vi "Track Rotation.vi"(8 "Angle Limiter":enum16{"90", "45", "15", "1"}(ring), 10 "Coord":cluster{dbl, dbl}, 11 "Point in":cluster{"x":dbl, "y":dbl, "th":dbl}) -> (3 "Point out":cluster{"x":dbl, "y":dbl, "th":dbl})   [LabVIEW 2018]
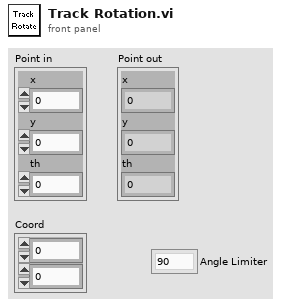
[diagram p1: front panel]
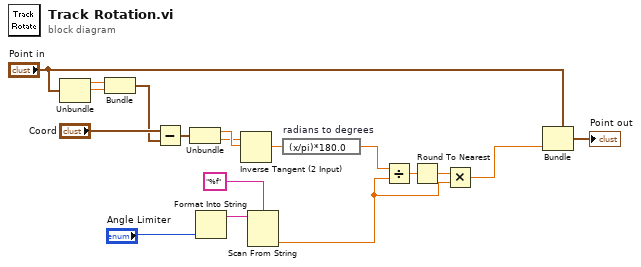
[diagram p0: block diagram]
diagram:
  n1 = Unbundle("Point in") -> ("x"=w15:dbl, "y"=w14:dbl)  [unwired: 1 out]
  n2 = Bundle("x"=w15, "y"=w14) -> (w13:cluster{"x":dbl, "y":dbl})  [unwired: 1 in]
  n3 = Subtract(x="Coord", y=w13) -> (x-y=w12:cluster{dbl, dbl})
  n4 = Unbundle(w12) -> (w11:dbl, w10:dbl)
  n5 = Format Into String("Angle Limiter") -> (resulting string=w5:string)  [unwired: 3 in, 1 out]
  n6 = Inverse Tangent (2 Input)(1:w11, 2:w10) -> (0:w9:dbl)
  n7 = Scan From String(format string="%f", input string=w5) -> (output 1=w1:dbl)  [unwired: 3 in, 3 out]
  n8 = expression code="(x/pi)*180.0" "radians to degrees"(w9) -> (w3:dbl)
  n9 = Divide(x=w3, y=w1) -> (x/y=w8:dbl)
  n10 = Round To Nearest(number=w8) -> (nearest integer value=w7:dbl)
  n11 = Multiply(x=w7, y=w1) -> (x*y=w2:dbl)
  n12 = Bundle(cluster="Point in", "th"=w2) -> (→"Point out":cluster{"x":dbl, "y":dbl, "th":dbl})  [unwired: 2 in]
